vi "text2pdf.vi"(8 "error in (no error)":errorcluster caption="错误输入（无错误）", 9 "Text":string caption="文本", 10 "File Path":path, 11 "PDF Filename":string="test.pdf") -> (0 "error out":errorcluster caption="错误输出")   [LabVIEW 2022 SP3]
uses:
  <vilib>/Utility/NIReport.llb/Report Type.ctl
  <vilib>/Utility/NIReport.llb/Append Report Text (str wrap).vi
  <vilib>/Utility/NIReport.llb/NI_report.lvclass
  <vilib>/Utility/NIReport.llb/NI_ReportGenerationCore.lvlib
  <vilib>/Utility/NIReport.llb/Word/NI_Word.lvclass
  <vilib>/Utility/NIReport.llb/Excel/NI_Excel.lvclass
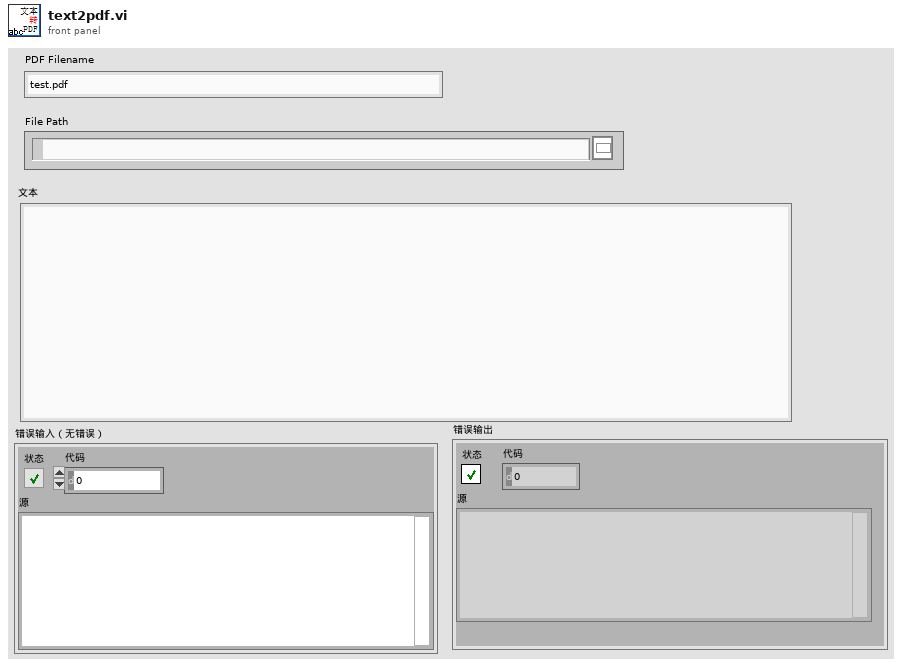
[diagram p1: front panel]
types:
  T1 = cluster{"Charset (-1)":i16, "Weight (-1)":i16, "Name":string, "Size":string}
  T2 = cluster{"Italic":enum16{"Italic Unchanged", "Italic On", "Italic Off"}, "Strike Through":enum16{"Strike Through Unchanged", "Strike Through On", "Strike Through Off"}, "Underline":enum16{"Underline Unchanged", "Underline On", "Underline Off"}, "Bold":enum16{"Bold Unchanged", "Bold On", "Bold Off"}}
  T3 = enum16{"maximized", "minimized", "normal", "no change"}
  T4 = typedef "NI_ReportGenerationCore.lvlib/Report Type.ctl" = enum16{"HTML", "Word", "Excel"}
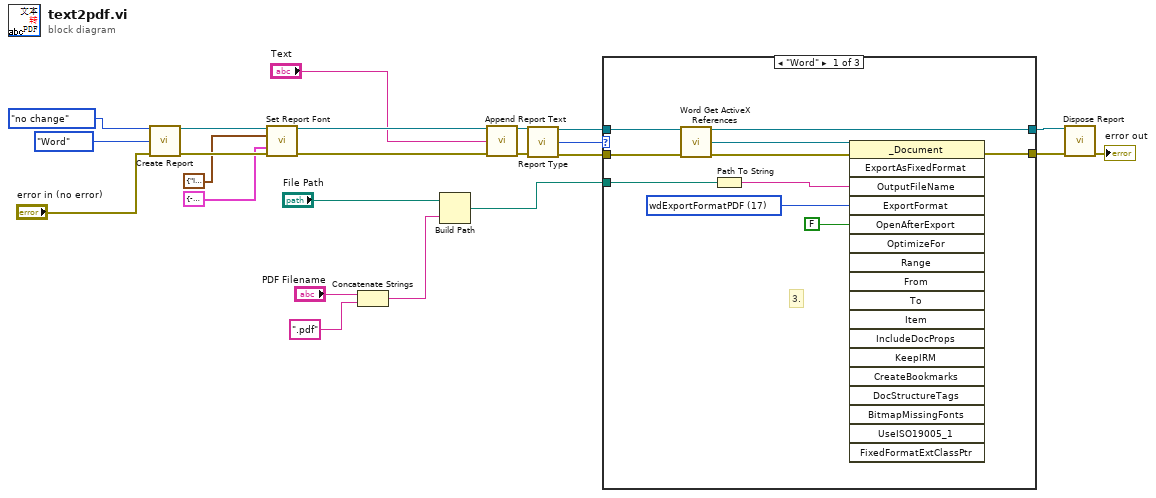
[diagram p0: block diagram]
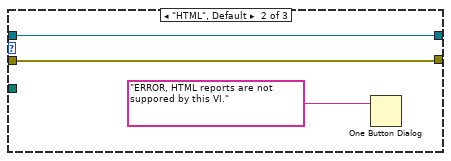
[diagram p2: hidden frame]
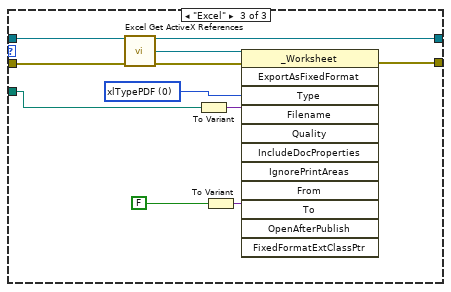
[diagram p3: hidden frame]
diagram:
  n1 = call <vilib>:"Create Report.vi"("window state (normal)"=T3."no change", "report type"=Report_Type."Word", "error in (no error)"="error in (no error)") -> ("report out"=w11:refnum<class "NI_report.lvclass">, "error out"=w12:errorcluster)  [unwired: 11 in]
  n2 = call-dynamic "Set Report Font.vi"("report in"=w11, "text options"=T2 {"Italic"=enum."Italic Unchanged", "Strike Through"=enum."Strike Through Unchanged", "Underline"=enum."Underline Unchanged", "Bold"=enum."Bold Unchanged"}, "font settings"=T1 {"Charset (-1)"=-1, "Weight (-1)"=-1, "Name"="", "Size"=" "}, "error in (no error)"=w12) -> ("report out"=w13:refnum<class "NI_report.lvclass">, "error out"=w4:errorcluster)  [unwired: 9 in, 1 out]
  n3 = Concatenate Strings("PDF Filename", ".pdf" ("字符串")) -> (w23:string)
  n4 = Build Path(base path="File Path", name or relative path=w23) -> (appended path=w19:path)
  n5 = call-poly <vilib>:"Append Report Text.vi"("report in"=w13, "text"="Text", "error in (no error)"=w4) -> ("report out"=w22:refnum<class "NI_report.lvclass">, "error out"=w20:errorcluster)  [unwired: 9 in, 2 out]
  n6 = call-dynamic "Report Type.vi"("report in"=w22, "error in (no error)"=w20) -> ("report out"=w15:refnum<class "NI_report.lvclass">, "report type"=w17:T4, "error out"=w16:errorcluster)  [unwired: 11 in]
  n7 = case shown="\"Word\"" w17 {
    tunnel: w15 -> [w33 w36 w46]
    tunnel: w19 -> [w30 _ w38]
    tunnel: [w32 w36 w44] -> w18
    tunnel: w16 -> [w27 w34 w43]
    tunnel: [w25 w34 w41] -> w21
    frame "Word" {
      w28 = 17 items=["wdExportFormatPDF"=17, "wdExportFormatXPS"=18] ("ExportFormat")
      # "3."
      n8 = call <vilib>:"Word Get ActiveX References.vi"("report in"=w33, "error in (no error)"=w27) -> ("report out"=w32:refnum<class "NI_report.lvclass">, "Word._Document"=w31:refnum<k7>, "error out"=w26:errorcluster)  [unwired: 7 in, 4 out]
      n9 = Path To String(path=w30) -> (string=w29:string)
      n10 = invoke class="_Document" method="ExportAsFixedFormat"(reference=w31, error in=w26, "OutputFileName"=w29, "ExportFormat"=w28, "OpenAfterExport"=FALSE) -> (error out=w25:errorcluster)  [unwired: 13 in, 17 out]
    }
    frame "HTML", Default {
      n11 = One Button Dialog(message="ERROR, HTML reports are not suppored by this VI.") -> ()  [unwired: 1 in, 1 out]
    }
    frame "Excel" {
      w40 = 0 items=["xlTypePDF", "xlTypeXPS"] ("Type")
      n12 = call <vilib>:"Excel Get ActiveX References.vi"("report in"=w46, "error in (no error)"=w43) -> ("report out"=w44:refnum<class "NI_report.lvclass">, "Excel._Worksheet"=w47:refnum<k7>, "error out"=w42:errorcluster)  [unwired: 7 in, 4 out]
      n13 = To Variant(anything=w38) -> (Variant=w37:variant)
      n14 = To Variant(anything=FALSE) -> (Variant=w39:variant)
      n15 = invoke class="_Worksheet" method="ExportAsFixedFormat"(reference=w47, error in=w42, "Type"=w40, "Filename"=w37, "OpenAfterPublish"=w39) -> (error out=w41:errorcluster)  [unwired: 7 in, 11 out]
    }
  }
  n16 = call-dynamic "Dispose Report.vi"("report in"=w18, "error in (no error)"=w21) -> ("error out"=→"error out":errorcluster)  [unwired: 13 in]
